vi "Test Simple Arduino Program 1.vi"(8 "Error In":errorcluster) -> (0 "Error Out":errorcluster, 3 "concatenated string":string)   [LabVIEW 2014]
panel:
  in  "sketch name":string="out"
  out "standard error":string
  out "standard output":string
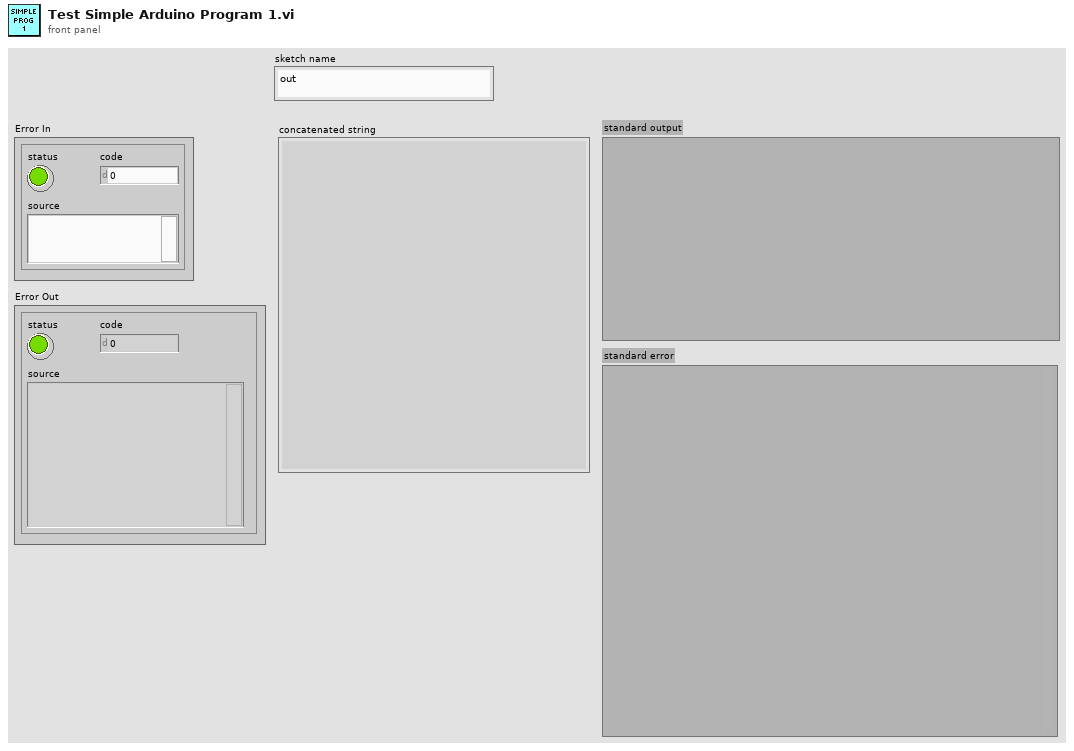
[diagram p1: front panel]
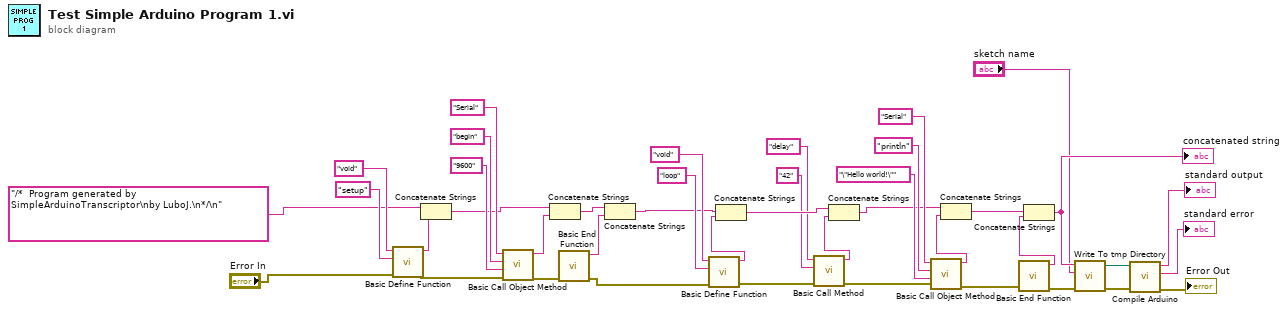
[diagram p0: block diagram]
diagram:
  n1 = call "Basic Define Function.vi"("Error In"="Error In", "name"="setup", "return type"="void") -> ("Error Out"=w33:errorcluster, "concatened string"=w39:string)  [unwired: 7 in]
  n2 = Concatenate Strings("/*  Program generated by SimpleArduinoTranscriptor\nby LuboJ.\n*/\n" ("string"), w39) -> (w28:string)
  n3 = call "Basic Call Object Method.vi"("Error In"=w33, "args"="9600", "method"="begin", "object name"="Serial") -> ("Error Out"=w34:errorcluster, "concatened string"=w29:string)  [unwired: 6 in]
  n4 = Concatenate Strings(w28, w29) -> (w30:string)
  n5 = call "Basic End Function.vi"("Error In"=w34) -> ("Error Out"=w9:errorcluster, "resulting string"=w38:string)  [unwired: 9 in]
  n6 = Concatenate Strings(w30, w38) -> (w22:string)
  n7 = call "Basic Define Function.vi"("Error In"=w9, "name"="loop", "return type"="void") -> ("Error Out"=w15:errorcluster, "concatened string"=w25:string)  [unwired: 7 in]
  n8 = Concatenate Strings(w22, w25) -> (w23:string)
  n9 = call "Basic Call Method.vi"("Error In"=w15, "args"="42", "method"="delay") -> ("Error Out"=w13:errorcluster, "concatened string"=w14:string)  [unwired: 7 in]
  n10 = Concatenate Strings(w23, w14) -> (w12:string)
  n11 = call "Basic Call Object Method.vi"("Error In"=w13, "args"="\"Hello world!\"", "method"="println", "object name"="Serial") -> ("Error Out"=w10:errorcluster, "concatened string"=w18:string)  [unwired: 6 in]
  n12 = Concatenate Strings(w12, w18) -> (w11:string)
  n13 = call "Basic End Function.vi"("Error In"=w10) -> ("Error Out"=w8:errorcluster, "resulting string"=w24:string)  [unwired: 9 in]
  n14 = Concatenate Strings(w11, w24) -> (w7:string)
  "concatenated string" <- w7
  n15 = call "Write To tmp Directory.vi"("error in (no error)"=w8, "sketch name"="sketch name", "arduino code"=w7) -> ("error out"=w6:errorcluster, "output file"=w5:path)  [unwired: 7 in]
  n16 = call "Compile Arduino.vi"("Error In"=w6, "input filename"=w5) -> ("Error Out"=→"Error Out":errorcluster, "standard error"=→"standard error":string, "standard output"=→"standard output":string)  [unwired: 7 in]
